vi "update mode in ui.vi"(8 "error in (no error)":errorcluster caption="에러 입력(에러 없음)", 10 "mode":T1, 11 "Haptic IC 입력":refnum<class "Haptic IC.lvclass">) -> (0 "error out":errorcluster caption="에러 출력", 3 "Haptic IC 출력":refnum<class "Haptic IC.lvclass">)   [LabVIEW 2020, in "Haptic IC.lvclass"]
uses:
  Haptic IC.lvclass
  Controls/(Ctrl)Mode.ctl
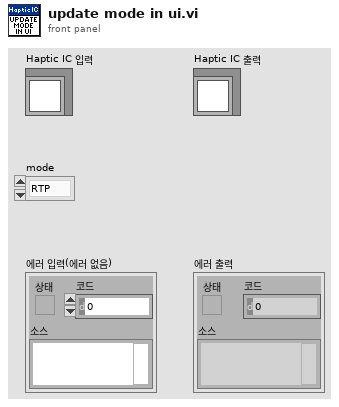
[diagram p1: front panel]
types:
  T1 = typedef "(Ctrl)Mode.ctl" = enum16{"RTP", "Memory"}
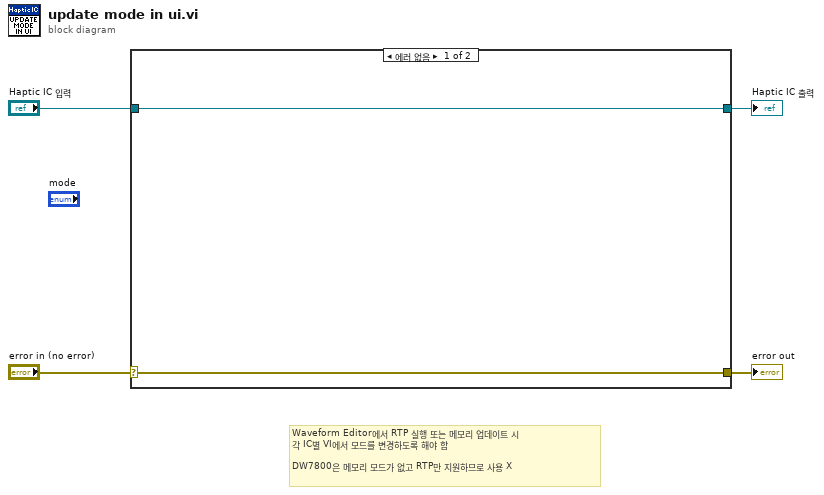
[diagram p0: block diagram]
diagram:
  # "Waveform Editor에서 RTP 실행 또는 메모리 업데이트 시\n각 IC별 VI에서 모드를 변경하도록 해야 함\n\nDW7800은 메모리 모드가 없고 RTP만 지원하므로 사용 X"
  n1 = case shown="에러 없음" "error in (no error)" {
    selector: "error in (no error)" -> [w5 w8]
    tunnel: [w5 w8] -> w3
    tunnel: [w6 w7] -> w1
    tunnel: "Haptic IC 입력" -> [w6 w7]
    frame No Error {
    }
    frame Error {
    }
  }
  "error out" <- w3
  "Haptic IC 출력" <- w1
